vi "Mean Gain and Phase.vi"(1 "Response":T2 {"Freq" format="%#.2f"; "Offset" format="%.3f"; "Gain" format="%.2f"; "Phase" format="%.1f"}, 2 "Stimulus":T2 {"Freq" format="%#.2f"; "Offset" format="%.3f"; "Gain" format="%.2f"; "Phase" format="%.1f"}) -> (0 "Gain and Phase out":T1 {"Phase SD" format="%.1f"; "Phase" format="%.1f"; "Gain SD" format="%.2f"; "Gain" format="%.2f"})   [LabVIEW 2013]
uses:
  Typedef - Sinusoidal Fit Coefficients.ctl
  Typedef - Gain and Phase.ctl
panel:
  # "Gain:"
  # "+/-"
  # "Phase:"
  # "+/-"
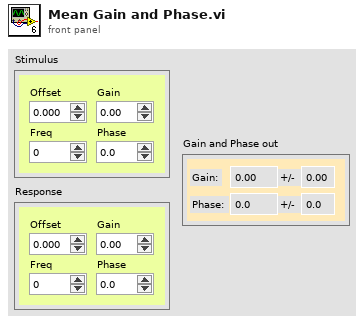
[diagram p1: front panel]
types:
  T1 = typedef "Typedef - Gain and Phase.ctl" = cluster{"Gain":dbl, "Gain SD":dbl, "Phase":dbl, "Phase SD":dbl}
  T2 = typedef "Typedef - Sinusoidal Fit Coefficients.ctl" = cluster{"Offset":dbl, "Gain":dbl, "Phase":dbl, "Freq":dbl}
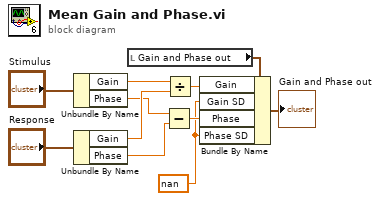
[diagram p0: block diagram]
diagram:
  w2 = nan
  n1 = Unbundle By Name("Stimulus") -> ("Gain"=w9:dbl, "Phase"=w5:dbl)
  n2 = Unbundle By Name("Response") -> ("Gain"=w8:dbl, "Phase"=w4:dbl)
  n3 = local read "Gain and Phase out"() -> (w7:T1)
  n4 = Subtract(x=w5, y=w4) -> (x-y=w3:dbl)
  n5 = Divide(x=w9, y=w8) -> (x/y=w6:dbl)
  n6 = Bundle By Name(cluster=w7, "Gain"=w6, "Gain SD"=w2, "Phase"=w3, "Phase SD"=w2) -> (→"Gain and Phase out":T1)
